vi "Dispose.vi"(8 "error in (no error)":errorcluster, 11 "Redis Client in":refnum<class "Redis Client.lvclass">) -> (0 "error out":errorcluster)   [LabVIEW 2019, in "Redis Client for LabVIEW.lvlib" / "Redis Client.lvclass"]
uses:
  Redis Client.lvclass
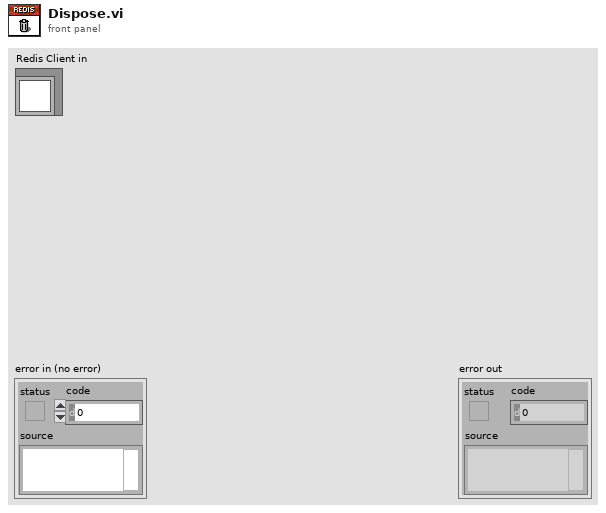
[diagram p1: front panel]
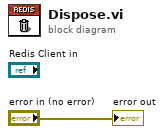
[diagram p0: block diagram]
diagram:
  "error out" <- "error in (no error)"
